vi "Ex2_Procesar.vi"(8 "error in (no error)":errorcluster, 10 "Señales":T2) -> (0 "error out":errorcluster, 2 "Señales Procesadas":T1)   [LabVIEW 2020]
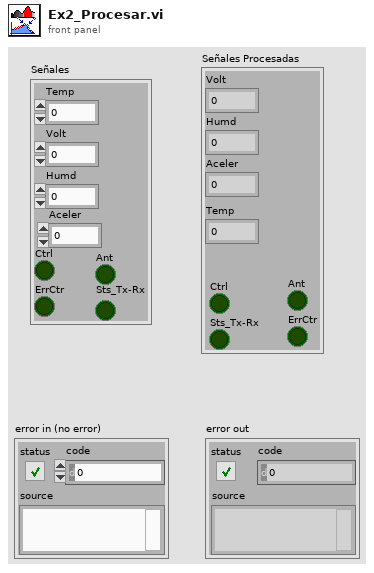
[diagram p1: front panel]
types:
  T1 = cluster{"Ant":bool, "ErrCtr":bool, "Volt":dbl, "Humd":dbl, "Aceler":dbl, "Ctrl":bool, "Sts_Tx-Rx":bool, "Temp":dbl}
  T2 = cluster{"Temp":dbl, "Volt":dbl, "Humd":dbl, "Ant":bool, "Ctrl":bool, "ErrCtr":bool, "Aceler":dbl, "Sts_Tx-Rx":bool}
  T3 = cluster{"D1":bool, "D3":bool, "A2":dbl, "A3":dbl, "A4":dbl, "D2":bool, "D4":bool, "A1":dbl}
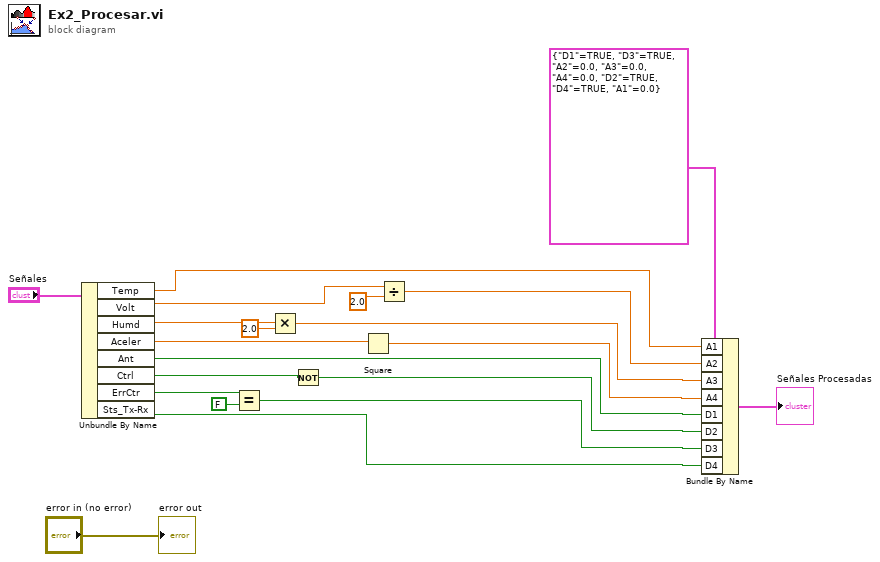
[diagram p0: block diagram]
diagram:
  n1 = Unbundle By Name("Señales") -> ("Temp"=w9:dbl, "Volt"=w18:dbl, "Humd"=w16:dbl, "Aceler"=w14:dbl, "Ant"=w5:bool, "Ctrl"=w13:bool, "ErrCtr"=w11:bool, "Sts_Tx-Rx"=w2:bool)
  n2 = Equal?(x=w11, y=FALSE) -> (x = y?=w3:bool)
  n3 = Multiply(x=w16, y=2.0) -> (x*y=w7:dbl)
  n4 = Not(x=w13) -> (.not. x?=w4:bool)
  n5 = Square(x=w14) -> (x^2=w6:dbl)
  n6 = Divide(x=w18, y=2.0) -> (x/y=w8:dbl)
  n7 = Bundle By Name(cluster=T3 {"D1"=TRUE, "D3"=TRUE, "A2"=0.0, "A3"=0.0, "A4"=0.0, "D2"=TRUE, "D4"=TRUE, "A1"=0.0}, "A1"=w9, "A2"=w8, "A3"=w7, "A4"=w6, "D1"=w5, "D2"=w4, "D3"=w3, "D4"=w2) -> (→"Señales Procesadas":T3)
  "error out" <- "error in (no error)"
